vi "Distancia.vi"(4 "error in (no error)":errorcluster, 6 "Unidad":enum16{"Cm", "mm", "Pulg"}(ring), 7 "Distancia":dbl) -> (0 "error out":errorcluster, 1 "pulg":dbl, 2 "cm":dbl, 3 "mm":dbl)   [LabVIEW 2020]
panel:
  in  "RETURN":bool
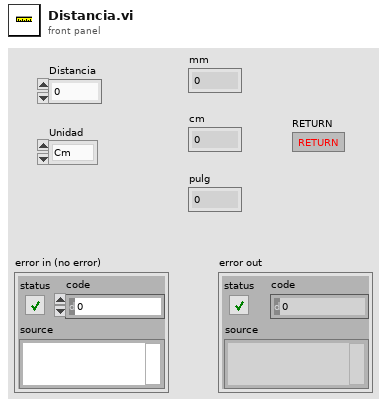
[diagram p1: front panel]
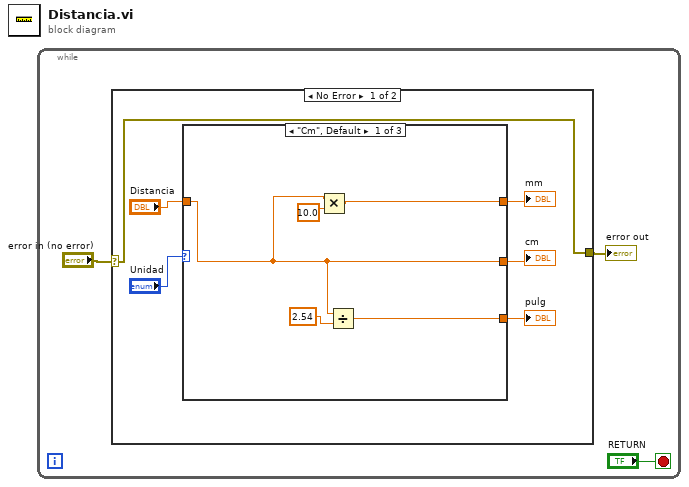
[diagram p0: block diagram]
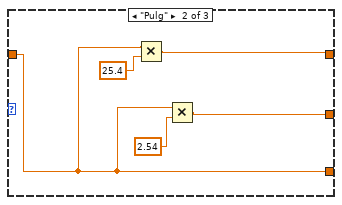
[diagram p2: hidden frame]
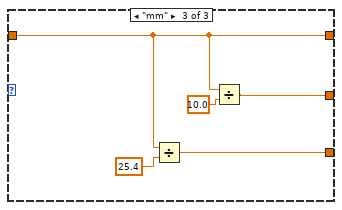
[diagram p3: hidden frame]
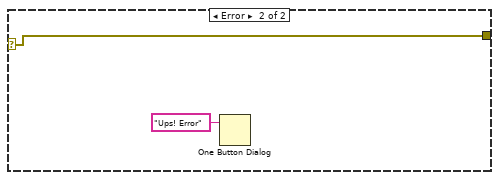
[diagram p4: hidden frame]
diagram:
  n1 = while {
    stop <- "RETURN" stop-if-true
    n2 = case shown="No Error" "error in (no error)" {
      selector: "error in (no error)" -> [w4 w25]
      tunnel: [w4 w25] -> w2
      frame No Error {
        n3 = case shown="\"Cm\", Default" "Unidad" {
          tunnel: [w11 w15 w21] -> w7
          tunnel: "Distancia" -> [w10 w16 w21]
          tunnel: [w10 w18 w23] -> w6
          tunnel: [w13 w16 w22] -> w5
          frame "Cm", Default {
            n4 = Multiply(x=w10, y=10.0) -> (x*y=w11:dbl)
            n5 = Divide(x=w10, y=2.54) -> (x/y=w13:dbl)
          }
          frame "Pulg" {
            n6 = Multiply(x=w16, y=25.4) -> (x*y=w15:dbl)
            n7 = Multiply(x=w16, y=2.54) -> (x*y=w18:dbl)
          }
          frame "mm" {
            n8 = Divide(x=w21, y=25.4) -> (x/y=w22:dbl)
            n9 = Divide(x=w21, y=10.0) -> (x/y=w23:dbl)
          }
        }
        "mm" <- w7
        "cm" <- w6
        "pulg" <- w5
      }
      frame Error {
        n10 = One Button Dialog(message="Ups! Error") -> ()  [unwired: 1 in, 1 out]
      }
    }
    "error out" <- w2
  }
